vi "SetOutputMixerFrequency.vi"(8 "error in (no error)":errorcluster, 9 "Output enabled":bool=TRUE, 10 "Output mixer fequency [MHz]":dbl, 11 "FpgaRef5782 in":refnum<class "FpgaRefx410.lvclass">) -> (0 "error out":errorcluster, 3 "FpgaRef5782 out":refnum<class "FpgaRefx410.lvclass">)   [LabVIEW 2025, in "FpgaRefx410.lvclass"]
uses:
  FpgaRefx410.lvclass
  FpgaRefx410.lvclass/FpgaRefx410.ctl
  <vilib>/rvi/interface/nirviReadWriteControl/nirviReadWriteControl.xnode
  x410 FPGA ref.ctl
  NiFpgaLv.dll
  <vilib>/Utility/error.llb/Error Cluster From Error Code.vi
  <vilib>/rvi/interface/Simulation/niFpgaSimulationCallBeginRW.vi
  <vilib>/rvi/errors/niLvFpgaAdjustHostInterfaceError.vi
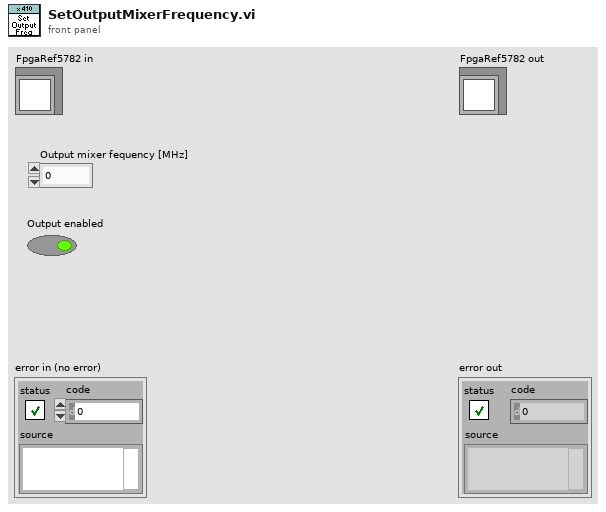
[diagram p1: front panel]
types:
  T1 = typedef "x410 FPGA ref.ctl" = refnum<k20>
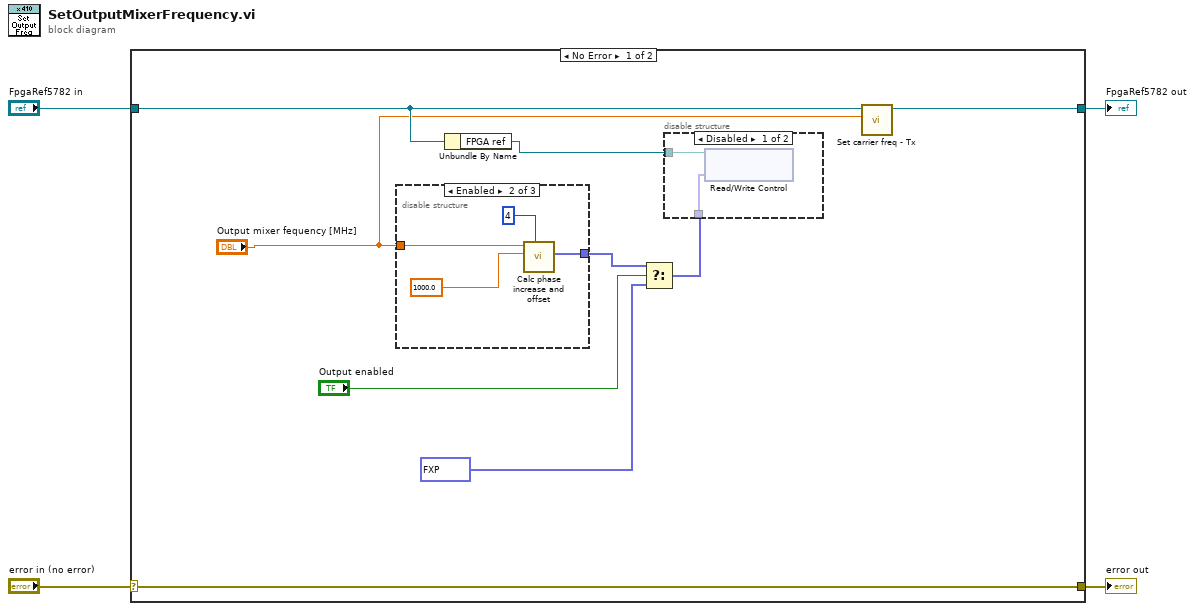
[diagram p0: block diagram]
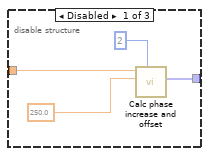
[diagram p3: hidden frame]
diagram:
  n1 = case shown="No Error" "error in (no error)" {
    selector: "error in (no error)" -> [w13 w25]
    tunnel: [w13 w25] -> w3
    tunnel: [w6 w24] -> w1
    tunnel: "FpgaRef5782 in" -> [w7 w24]
    frame No Error {
      n2 = disable-structure shown="Enabled" {
        disable-tunnel: [w17 w21 _] -> w10
        disable-tunnel: "Output mixer fequency [MHz]" -> [w16 w20 _]
        frame Disabled {
          n3 = call "Calc phase increase and offset.vi"("# of DDS"=2, "fclk (MHz)"=250.0 ("fclk (800MHz)"), "f_generated (MHz)"=w16) -> ("Phase out"=w17:fxp<+,64,64>[])  [unwired: 6 in, 2 out]
        }
        frame Enabled {
          n4 = call "Calc phase increase and offset.vi"("# of DDS"=4, "fclk (MHz)"=1000.0 ("fclk (800MHz)"), "f_generated (MHz)"=w20) -> ("Phase out"=w21:fxp<+,64,64>[])  [unwired: 6 in, 2 out]
        }
        frame Disabled {
        }
      }
      n5 = Unbundle By Name(w7) -> ("FPGA ref"=w8:T1)
      n6 = Select(t=w10, s="Output enabled", f=fxp<+,64,64>[] [0.0, 0.0, 0.0, 0.0, 0.0, 0.0, 0.0, 0.0, 0.0, 0.0, 0.0, 0.0, 0.0, 0.0, 0.0, 0.0]) -> (s? t:f=w9:fxp<+,64,64>[])
      n7 = disable-structure shown="Disabled" {
        disable-tunnel: w9 -> [w15 _]
        disable-tunnel: w8 -> [w14 _]
        frame Disabled {
          n8 = xnode "Read/Write Control"("FPGA VI Reference In"=w14, "Phase output"=w15) -> ()  [unwired: 1 in, 2 out]
        }
        frame Enabled {
        }
      }
      n9 = call-dynamic "Set carrier freq - Tx.vi"("Carrier freq [MHz]"="Output mixer fequency [MHz]", "FpgaRefx410 in"=w7) -> ("FpgaRefx410 out"=w6:refnum<class "FpgaRefx410.lvclass">)  [unwired: 8 in, 1 out]
    }
    frame Error {
    }
  }
  "error out" <- w3
  "FpgaRef5782 out" <- w1
